vi "Variant to Attribute.vi"(8 "Error In":errorcluster, 10 "Parameter":variant, 11 "Actor Framework:Message in":refnum<class>) -> (0 "Error Out":errorcluster, 3 "Actor Framework:Message out":refnum<class>)   [LabVIEW 2016]
doc: "(<B>Filename</B>: Actor Framework.lvlib:Message.lvclass:Variant to Attribute.vi)\n\nRead message attributes from parameter variant.\n\n<b>Attention:</b> This dynamic dispatch VI was added to the Message.lvclass in order to provide a mechnism to allow for generic parameter parsing. Refer to CS++LNA.lvlib:CS++LNAMessage.lvclass.Do.vi"
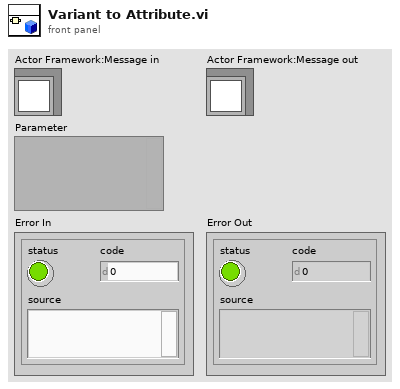
[diagram p1: front panel]
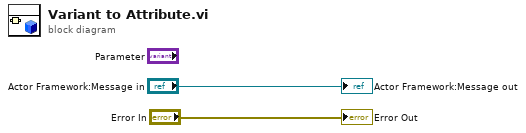
[diagram p0: block diagram]
diagram:
  "Error Out" <- "Error In"
  "Actor Framework:Message out" <- "Actor Framework:Message in"
